vi "Test.vi"() -> ()   [LabVIEW 2019]
uses:
  grpc-lvsupport/Message Metadata.ctl
  grpc-lvsupport/Message Element Metadata.ctl
  grpc-lvsupport/Message Element Type.ctl
  grpc-lvsupport/grpc-lvsupport.lvlib
panel:
  out "error out":errorcluster
  out "Listening Port":i32
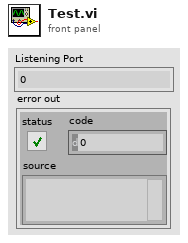
[diagram p1: front panel]
types:
  T1 = typedef "grpc-lvsupport.lvlib/Message Metadata.ctl" = cluster{"Version":i32, "Name":string, "Type Url":string, "Elements":T2[], "Has Oneof":bool}
  T2 = typedef "grpc-lvsupport.lvlib/Message Element Metadata.ctl" = cluster{"Field Name":string, "Embedded Message Name":string, "Protobuf Index":i32, "MessageElementType":T3, "Repeated":bool, "Is in Oneof":bool, "Oneof Container Name":string}
  T3 = typedef "grpc-lvsupport.lvlib/Message Element Type.ctl" = enum32{"Int32Value", "FloatValue", "DoubleValue", "BoolValue", "StringValue", "MessageValue", "Int64Value", "UInt32Value", "UInt64Value", "EnumValue", "Bytes", "Fixed64", "Fixed32", "SFixed64", "SFixed32", "SInt64", "SInt32"}
  T4 = typedef "grpc-lvsupport.lvlib/grpcId.ctl" = u64
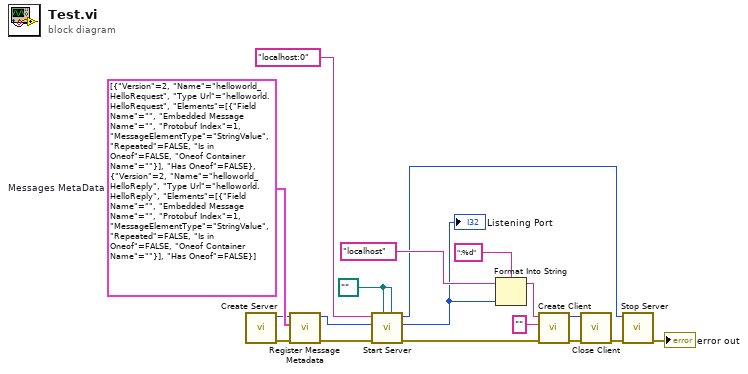
[diagram p0: block diagram]
diagram:
  w7 = T1[] [{"Version"=2, "Name"="helloworld_HelloRequest", "Type Url"="helloworld.HelloRequest", "Elements"=[{"Field Name"="", "Embedded Message Name"="", "Protobuf Index"=1, "MessageElementType"=enum."StringValue", "Repeated"=FALSE, "Is in Oneof"=FALSE, "Oneof Container Name"=""}], "Has Oneof"=FALSE}, {"Version"=2, "Name"="helloworld_HelloReply", "Type Url"="helloworld.HelloReply", "Elements"=[{"Field Name"="", "Embedded Message Name"="", "Protobuf Index"=1, "MessageElementType"=enum."StringValue", "Repeated"=FALSE, "Is in Oneof"=FALSE, "Oneof Container Name"=""}], "Has Oneof"=FALSE}]  # Messages MetaData
  w18 = path "" ("Server Certificate File (.crt)")
  n1 = call "Create Server.vi"() -> ("error out"=w4:errorcluster, "gRPCid out"=w5:T4)  [unwired: 10 in]
  n2 = call "Register Message Metadata.vi"("error in"=w4, "Messages"=w7, "gRPCid in"=w5) -> ("error out"=w3:errorcluster, "gRPCid out"=w6:T4)  [unwired: 7 in]
  n3 = call "Start Server.vi"("Server Key File (.key)"=w18, "Server Certificate File (.crt)"=w18, "error in"=w3, "gRPCid server in"=w6, "Server Address"="localhost:0") -> ("error out"=w2:errorcluster, "Listening Port"=w15:i32, "gRPCid server out"=w1:T4)  [unwired: 4 in]
  "Listening Port" <- w15
  n4 = Format Into String(format string=":%d", initial string="localhost" ("address"), w15) -> (resulting string=w13:string)  [unwired: 1 in, 1 out]
  n5 = call "Create Client.vi"("error in"=w2, "certificatePath"="", "address"=w13) -> ("error out"=w11:errorcluster, "ClientID out"=w12:T4)  [unwired: 7 in]
  n6 = call "Close Client.vi"("error in"=w11, "ClientID in"=w12) -> ("error out"=w9:errorcluster)  [unwired: 9 in]
  n7 = call "Stop Server.vi"("error in"=w9, "gRPCid server in"=w1) -> ("error out"=→"error out":errorcluster)  [unwired: 9 in]
